vi "GetChannelMask.vi"(1 "ChainNumber":u8) -> (0 "ChainMask":u8)   [LabVIEW 2020, in "ArduinoSerialBling.lvlib"]
uses:
  Documents/Robotics/swerve-template/Swerve Robot Project Template/LEDs/Implementation/ArduinoSerialBling.lvlib
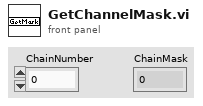
[diagram p1: front panel]
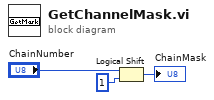
[diagram p0: block diagram]
diagram:
  n1 = Logical Shift(y="ChainNumber", x=u8 1) -> (x << y=→"ChainMask":u8)
